vi "Calc Distance Array.vi"(11 "Wheel info":T1={"Names"=[], "Relative Position"=[0, 10000, 17000, 25000, 33000, 40000], "Wheel Name"="", "Size"=0}) -> (3 "Distances":i32[](array[numeric]))   [LabVIEW 2022 SP3, in "FW Arduino Control.lvclass"]
uses:
  FW Arduino Control.lvclass
  Filter Wheel Object/Filter Wheel Details.ctl
  FW Arduino Control.lvclass/FW Arduino Control.ctl
  Filter Wheel Object/Filter Wheel.lvclass
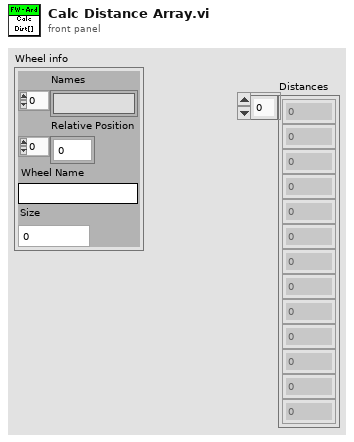
[diagram p1: front panel]
types:
  T1 = typedef "Filter Wheel.lvclass/Filter Wheel Details.ctl" = cluster{"Names":string[], "Relative Position":i32[], "Wheel Name":string, "Size":i32}
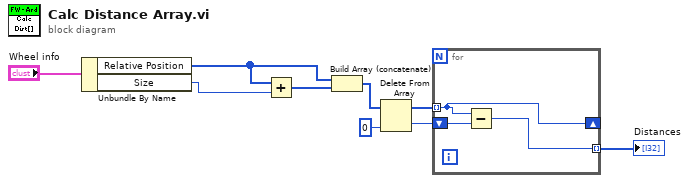
[diagram p0: block diagram]
diagram:
  n1 = Unbundle By Name("Wheel info") -> ("Relative Position"=w4:i32[], "Size"=w2:i32)
  n2 = Add(x=w4, y=w2) -> (x+y=w3:i32[])
  n3 = Build Array (concatenate)(w4, w3) -> (w9:i32[])
  n4 = Delete From Array(array=w9, index=0) -> (deleted portion=w7:i32, array with subset deleted=w8:i32[])  [unwired: 1 in]
  n5 = for {
    tunnel: w8 -> [w11] mode=indexing
    shift-right: [w11] -> _
    shift-left: w7 -> [w12]
    tunnel: [w10] -> w5 mode=indexing
    n6 = Subtract(x=w11, y=w12) -> (x-y=w10:i32)
  }
  "Distances" <- w5
